vi "Distance Sensor PWM TEST.vi"() -> ()   [LabVIEW 2017]
doc: "This example shows how to use the MaxBotix LV-MaxSonar-EZ1 Sonar Range Finder MB1010. It will display the distance from the sensor in inches.\n\nThis example expects a USB cable connected from your development PC to the Type B USB Jack (next to the power input) on the roboRIO."
uses:
  <vilib>/Rock Robotics/WPI/Ultrasonic/WPI_SonarMB1010DigitalGetRange.vi
  <vilib>/Rock Robotics/WPI/Ultrasonic/WPI_SonarMB1010DigitalClose.vi
  <vilib>/Rock Robotics/SystemInterfaces/DIO/FPGA_DIOChannel.ctl
panel:
  out "distance":dbl(slide)=125.0 scale=0.0..250.0 scale format="%3d"
  in  "Scaling factor (s/in)":dbl=0.000147
  in  "DIO Channel":T1=enum."DIO 5"
  in  "stop":bool
  # "Set these inputs before running."
  # "This can be set while runnning."
  # "This shows wiring for a MaxBotix LV-MaxSonar-EZ1 Sonar Range Finder MB1010."
  # "EZ1 MB1010"
  # "EZ1 MB1010\nGND (black wire)------\n+5 (red wire)----------\nPW (white wire)-------"
  # "roboRIO\nDIO-5 \nDIO-5  V\nDIO-5  S"
  # "Output information."
  # "EZ1"
  # "inches"
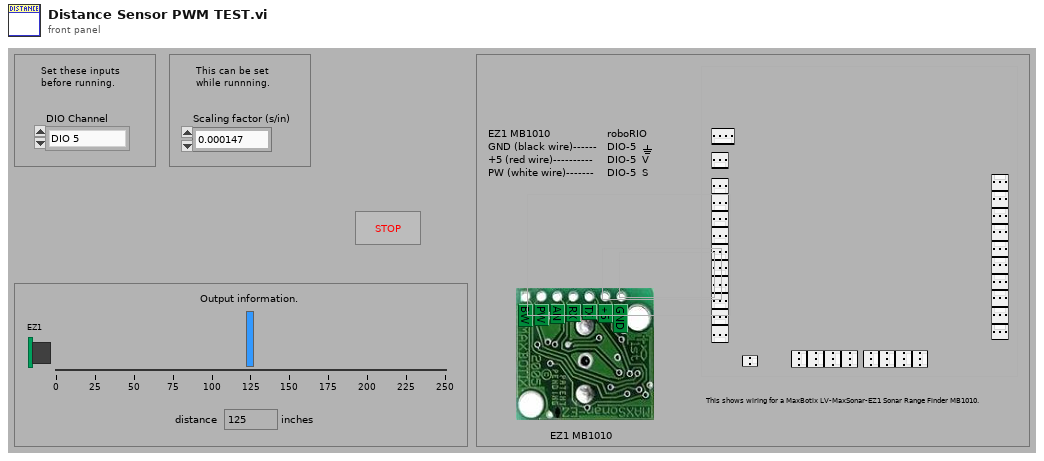
[diagram p1: front panel]
types:
  T1 = typedef "FPGA_DIOChannel.ctl" = enum8{"DIO 0", "DIO 1", "DIO 2", "DIO 3", "DIO 4", "DIO 5", "DIO 6", "DIO 7", "DIO 8", "DIO 9", "DIO MXP 0", "DIO MXP 1", "DIO MXP 2", "DIO MXP 3", "DIO MXP 4", "DIO MXP 5", "DIO MXP 6", "DIO MXP 7", "DIO MXP 8", "DIO MXP 9", "DIO MXP 10", "DIO MXP 11", "DIO MXP 12", "DIO MXP 13", "DIO MXP 14", "DIO MXP 15", "SPI Port CS1", "SPI Port CS2", "SPI Port CS3", "SPI Port MISO", "SPI Port MOSI", "Invalid"}
  T2 = typedef "WPI_SonarMB1010DigitalDeviceRef.ctl" = cluster{"CounterDevRef":T3, "Scaling factor (s/in)":dbl}
  T3 = typedef "WPI_CounterDevRef.ctl" = cluster{"DevStatus":errorcluster, "CntIndex":T4}
  T4 = typedef "FPGA_CounterCtrSystemIndex.ctl" = enum8{"Ctr 0", "Ctr 1", "Ctr 2", "Ctr 3", "Ctr 4", "Ctr 5", "Ctr 6", "Ctr 7", "Invalid"}
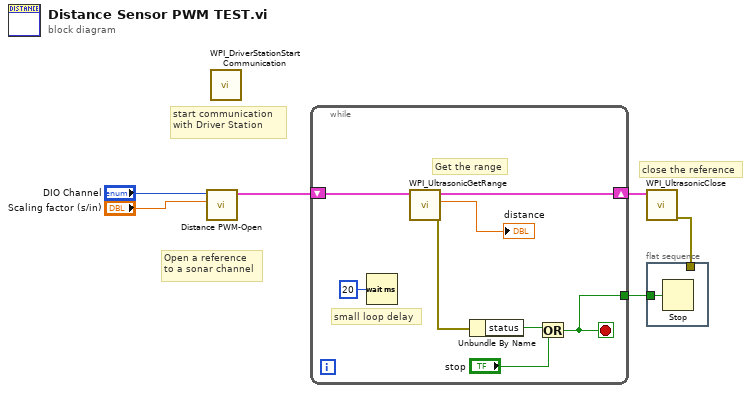
[diagram p0: block diagram]
diagram:
  # "start communication with Driver Station"
  # "close the reference"
  # "Open a reference\nto a sonar channel"
  n1 = call "Distance PWM-Open.vi"(10:"Scaling factor (s/in)", "DIO Channel"="DIO Channel") -> ("SonarMB1010DigitalDevRef"=w1:T2)  [unwired: 8 in, 1 out]
  n2 = call <vilib>:"WPI_DriverStationStart Communication.vi"() -> ()  [unwired: 2 in, 10 out]
  n3 = while {
    shift-right: [w14] -> w5
    shift-left: w1 -> [w8]
    tunnel: [w11] -> w6
    stop <- w11 stop-if-true
    # "small loop delay"
    # "Get the range"
    n4 = Wait (ms)(milliseconds to wait=u32 20) -> ()  [unwired: 1 out]
    n5 = call-poly <vilib>:"WPI_UltrasonicGetRange.vi"("SonarMB1010DigitalDevRef"=w8) -> ("error out"=w10:errorcluster, "Distance"=→"distance":dbl, "SonarMB1010DigitalDevRef"=w14:T2)  [unwired: 8 in]
    n6 = Unbundle By Name(w10) -> ("status"=w12:bool)
    n7 = Or(x=w12, y="stop") -> (x .or. y?=w11:bool)
  }
  n8 = call-poly <vilib>:"WPI_UltrasonicClose.vi"("SonarMB1010DigitalDevRef"=w5) -> ("error out"=w4:errorcluster)  [unwired: 10 in]
  n9 = flat-sequence {
    tunnel: w6 -> [w15]
    tunnel: w4 -> [_]
    frame #0 {
      n10 = Stop(stop? (T)=w15) -> ()
    }
  }
